vi "Wrap values off neighbours.vi"(11 "Array in":u32[][][](array[numeric])) -> (3 "Array out":u32[][][](array[numeric]))   [LabVIEW 2013]
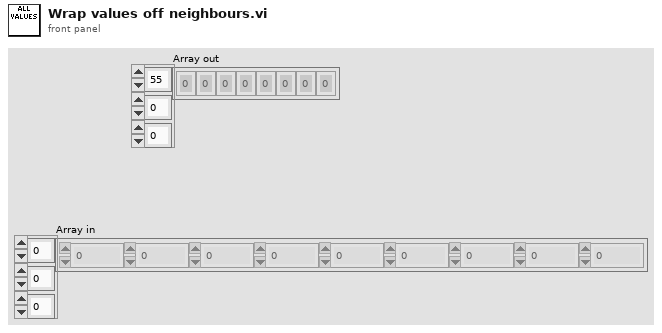
[diagram p1: front panel]
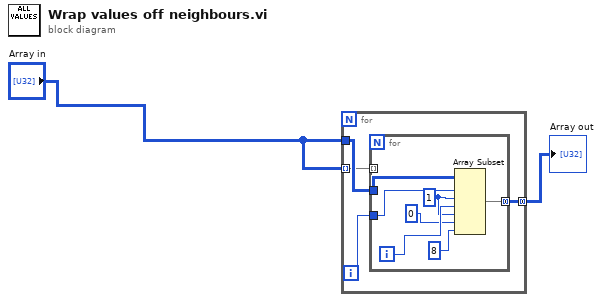
[diagram p0: block diagram]
diagram:
  n1 = for {
    tunnel: "Array in" -> [w6]
    tunnel: "Array in" -> [w5] mode=indexing
    tunnel: [w3] -> w2 mode=concatenating
    i -> [w4]
    n2 = for {
      tunnel: w6 -> [w13]
      tunnel: w5 -> [_] mode=indexing
      tunnel: w4 -> [w12]
      tunnel: [w7] -> w3 mode=concatenating
      i -> [w11]
      w8 = 1 ("length")
      n3 = Array Subset(array=w13, index (dim 0)=w12, length (dim 0)=w8, index (dim 1)=w11, length (dim 1)=w8, index (dim 2)=0 ("length"), length (dim 2)=8 ("length")) -> (w7:u32[][][])
    }
  }
  "Array out" <- w2
